vi "OverlayArc.vi"   [LabVIEW 2024, in "OpenLvVision_Overlays.lvlib"]
doc: "Overlays an line on top of an image."
uses:
  OpenLvVision_Overlays.lvlib
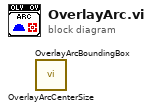
[diagram p0: block diagram]
diagram:
  n1 = call "OverlayArcCenterSize.vi"() -> ()  [unwired: 14 in, 2 out]
  n2 = call "OverlayArcBoundingBox.vi"() -> ()  [unwired: 10 in, 2 out]
